vi "Resize VI FP in place.vi"(6 "Target in":refnum<vi>, 7 "VI reference in":refnum<vi>, 8 "error in (no error)":errorcluster, 9 "Height":u32, 10 "Width":u32, 11 "Position":T1={"Left"=2147483647, "Top"=2147483647}) -> (0 "error out":errorcluster, 3 "VI reference out":refnum<vi>, 4 "Target out":refnum<vi>)   [LabVIEW 2020]
uses:
  <vilib>/Utility/miscctls.llb/LVPositionTypeDef.ctl
  <vilib>/Utility/miscctls.llb/LVRectTypeDef.ctl
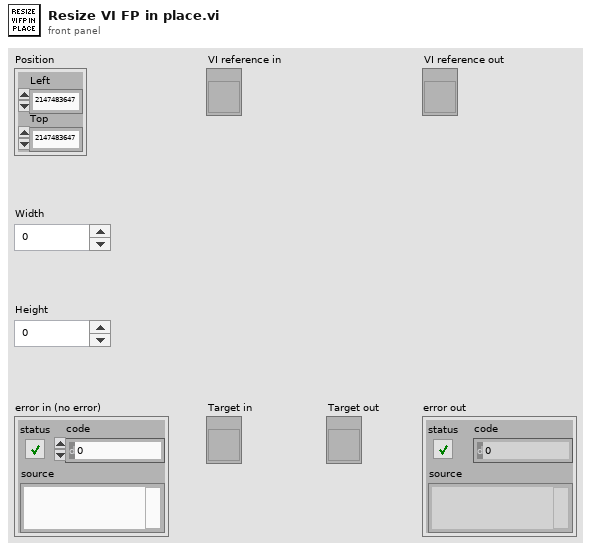
[diagram p1: front panel]
types:
  T1 = typedef "LVPositionTypeDef.ctl" = cluster{"Left":i32, "Top":i32}
  T2 = typedef "LVRectTypeDef.ctl" = cluster{"Left":i16, "Top":i16, "Right":i16, "Bottom":i16}
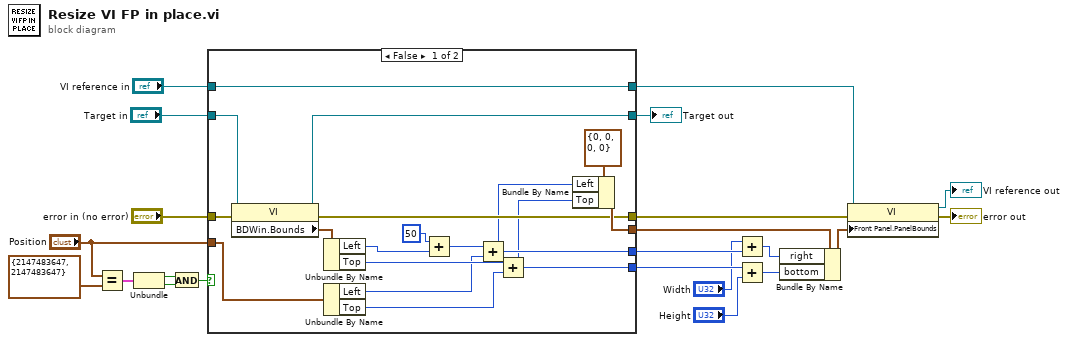
[diagram p0: block diagram]
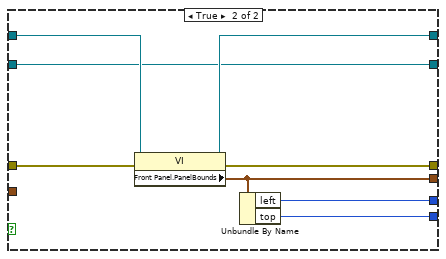
[diagram p2: hidden frame]
diagram:
  n1 = Equal?(x="Position", y=T1 {"Left"=2147483647, "Top"=2147483647} ("blah")) -> (x = y?=w7:cluster{"Left":bool, "Top":bool})
  n2 = Unbundle(w7) -> ("Left"=w6:bool, "Top"=w5:bool)
  n3 = And(x=w6, y=w5) -> (x .and. y?=w4:bool)
  n4 = case shown="False" w4 {
    tunnel: [w36 w47] -> w21
    tunnel: [w27 w46] -> w20
    tunnel: [w37 w45] -> w19
    tunnel: [w31 w44] -> w18
    tunnel: [w29 w43] -> w16
    tunnel: "VI reference in" -> [w27 w42]
    tunnel: "error in (no error)" -> [w35 w41]
    tunnel: "Position" -> [w39 _]
    tunnel: "Target in" -> [w28 w40]
    tunnel: [w26 w40] -> w1
    frame False {
      n5 = property class="VI"(reference=w28, error in=w35) -> (reference out=w26:refnum<vi>, error out=w36:errorcluster, "BDWin.Bounds"=w34:T2)
      n6 = Unbundle By Name(w34) -> ("Left"=w25:i16, "Top"=w33:i16)
      n7 = Unbundle By Name(w39) -> ("Left"=w32:i32, "Top"=w30:i32)
      n8 = Add(x=i16 50, y=w25) -> (x+y=w24:i16)
      n9 = Add(x=w24, y=w32) -> (x+y=w31:i32)
      n10 = Add(x=w33, y=w30) -> (x+y=w29:i32)
      n11 = Bundle By Name(cluster=T2 {"Left"=0, "Top"=0, "Right"=0, "Bottom"=0} ("Front Panel Window:Panel Bounds"), "Left"=w31, "Top"=w29) -> (w37:T2)
    }
    frame True {
      n12 = property on="Property Node" class="VI"(reference=w42, error in=w41) -> (reference out=w46:refnum<vi>, error out=w47:errorcluster, "Front Panel.PanelBounds"=w45:T2)
      n13 = Unbundle By Name(w45) -> ("left"=w44:i16, "top"=w43:i16)
    }
  }
  "Target out" <- w1
  n14 = Add(x="Width", y=w18) -> (x+y=w17:u32)
  n15 = Add(x=w16, y="Height") -> (x+y=w15:u32)
  n16 = Bundle By Name(cluster=w19, "right"=w17, "bottom"=w15) -> (w22:T2)
  n17 = property on="Property Node" class="VI"(reference=w20, error in=w21, "Front Panel.PanelBounds"=w22) -> (reference out=→"VI reference out":refnum<vi>, error out=→"error out":errorcluster)
